vi "Determine Column Constraints.vi"(8 "error in (no error)":errorcluster, 11 "Composed Column Factory in":refnum<class "Composed Column Factory.lvclass">) -> (0 "error out":errorcluster, 2 "Column Constraints":refnum<class "Constraint Manager.lvclass">, 3 "Composed Column Factory out":refnum<class "Composed Column Factory.lvclass">)   [LabVIEW 2020, in "Composed Columns.lvlib" / "Composed Column Factory.lvclass"]
uses:
  Composed Column Factory.lvclass
  Check Manager/Constraint Manager.lvclass
  Composed Column Factory.lvclass/Composed Column Factory.ctl
  Unique/Unique.lvclass
  C:/Users/User/Desktop/Raman Program/Database OOP/source/Database OOP/Column Libraries/Check/Constraint.lvclass
  Autoincrement/Autoincrement.lvclass
  Basic Columns/Column Configuration/Basic Column Configuration Class/Column Configuration.lvclass
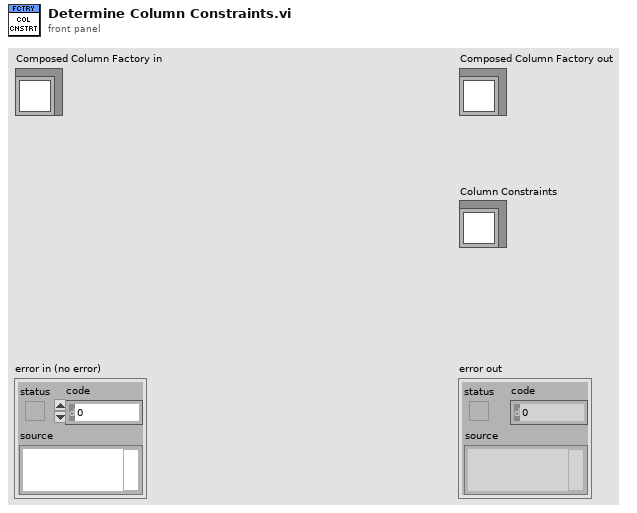
[diagram p1: front panel]
types:
  T1 = typedef "Database Interfaces.lvlib/Database data type.ctl" = enum16{"Undefined", "String", "Long (I32)", "Single (SGL)", "Double (DBL)", "Date/Time", "Binary"}
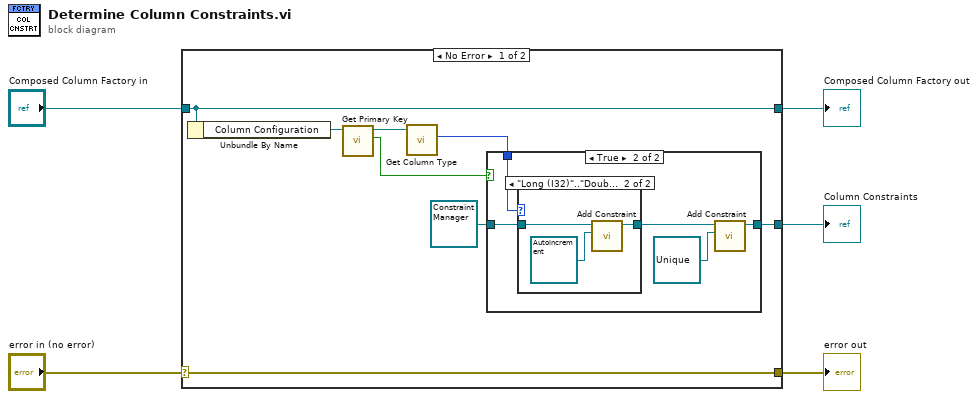
[diagram p0: block diagram]
diagram:
  n1 = case shown="No Error" "error in (no error)" {
    selector: "error in (no error)" -> [w13 w25]
    tunnel: [w13 w25] -> w4
    tunnel: [w10 w24] -> w2
    tunnel: "Composed Column Factory in" -> [w10 w24]
    tunnel: [w11 _] -> w1
    frame No Error {
      n2 = Unbundle By Name(w10) -> ("Column Configuration"=w9:refnum<class "Column Configuration.lvclass">)
      n3 = call-dynamic "Get Primary Key.vi"("Basic Column Configuration in"=w9) -> ("Is a PK?"=w8:bool, "Basic Column Configuration out"=w6:refnum<class "Column Configuration.lvclass">)  [unwired: 8 in, 1 out]
      n4 = call-dynamic "Get Column Type.vi"("Basic Column Configuration in"=w6) -> ("Column Type"=w7:T1)  [unwired: 8 in, 2 out]
      n5 = case shown="True" w8 {
        tunnel: w7 -> [_ w19]
        tunnel: refnum<class "Constraint Manager.lvclass"> refnum ("Composed Columns.lvlib:Constraint Manager.lvclass") -> [w14 w18]
        tunnel: [w14 w15] -> w11
        frame False {
        }
        frame True {
          n6 = case shown="\"Long (I32)\"..\"Double (DBL)\"" w19 {
            tunnel: w18 -> [w20 w23]
            tunnel: [w20 w22] -> w17
            frame Default {
            }
            frame "Long (I32)".."Double (DBL)" {
              n7 = call "Add Constraint.vi"("Check"=refnum<class "Autoincrement.lvclass"> refnum ("Composed Columns.lvlib:Autoincrement.lvclass"), "Check Manager in"=w23) -> ("Check Manager out"=w22:refnum<class "Constraint Manager.lvclass">)  [unwired: 8 in, 1 out]
            }
          }
          n8 = call "Add Constraint.vi"("Check"=refnum<class "Unique.lvclass"> refnum ("Composed Columns.lvlib:Unique.lvclass"), "Check Manager in"=w17) -> ("Check Manager out"=w15:refnum<class "Constraint Manager.lvclass">)  [unwired: 8 in, 1 out]
        }
      }
    }
    frame Error {
    }
  }
  "error out" <- w4
  "Composed Column Factory out" <- w2
  "Column Constraints" <- w1
